vi "Ic distribution Contour_KEPCO.vi"() -> ()   [LabVIEW 2021]
uses:
  global.vi
  <vilib>/Utility/file.llb/Write Delimited Spreadsheet (DBL).vi
panel:
  in  "Field Output Channel":i32=1
  in  "NI-DAQ Device Number":i32=1
  in  "Field Read Channel":tag="Dev1/ai2"
  in  "Scale factor":dbl=34.3054
  out "Current Field mT":dbl=-2.9845698000000005
  in  "Ramp Rate V per Sec":dbl=0.001
  in  "Frequency Hz":dbl=50.0
  in  "Vmax":dbl=2.0
  out "Current Field V":dbl=-0.08700000000000002
  out "error out":errorcluster
  in  "Name":string="book14"
  in  "Contour plot folder":path=path "\\\\ad.uillinois.edu\\engr/mrl-dvh-research/Guang Yue/data/Contour plot"
  in  "End field V":dbl=-0.087 format="%#_13g"
  in  "Field step V":dbl=-0.0005 format="%#_13g"
  in  "Start field V":dbl=0.175 format="%#_13g"
  # "Set default of Ic VI before Run."
  # "Max 5mV/s"
  # "V_Field*Scale=mT"
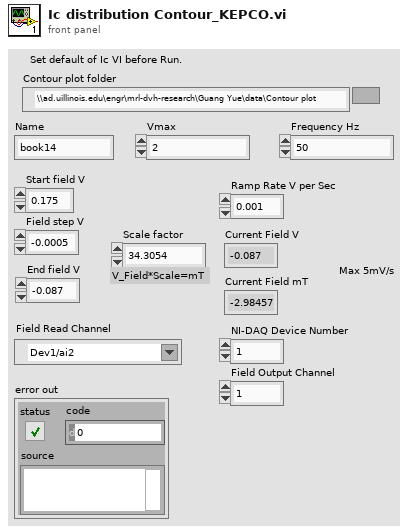
[diagram p1: front panel]
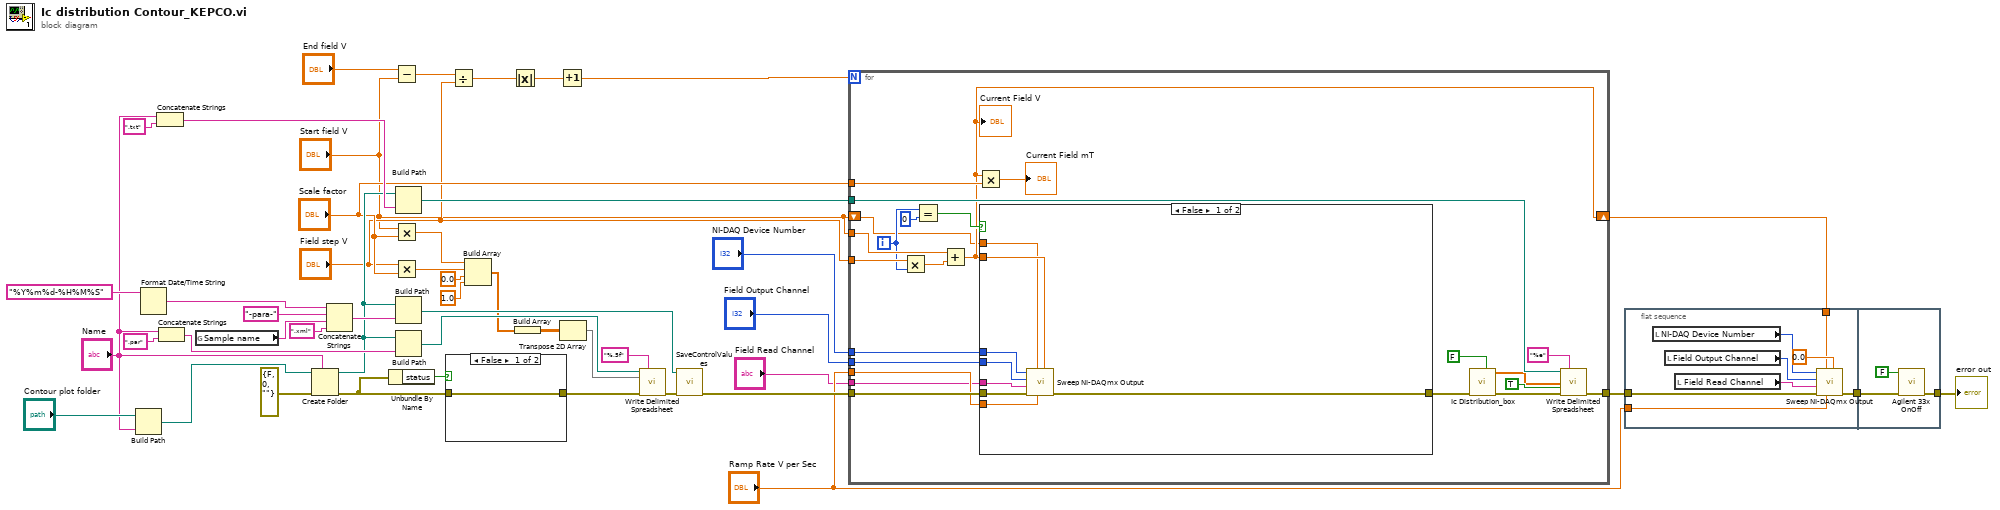
[diagram p0: block diagram]
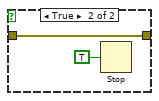
[diagram p2: hidden frame]
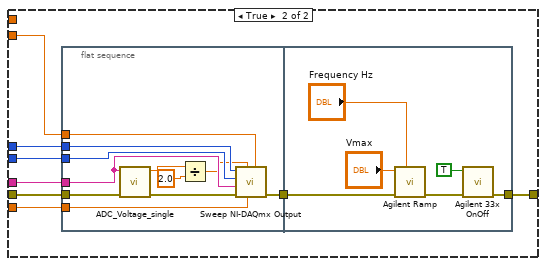
[diagram p3: hidden frame]
diagram:
  n1 = Build Path(base path="Contour plot folder", name or relative path="Name") -> (appended path=w24:path)
  n2 = Format Date/Time String(time format string (%c)="%Y%m%d-%H%M%S") -> (date/time string=w18:string)  [unwired: 2 in]
  n3 = Concatenate Strings("Name", ".txt" ("string")) -> (w28:string)
  n4 = Concatenate Strings("Name", ".par" ("string")) -> (w35:string)
  n5 = global read "global.vi" "Sample name"() -> (w17:string)
  n6 = Create Folder(prompt (Create Folder)="Name", path (use dialog)=w24, error in=errorcluster {"status"=FALSE, "code"=0, "source"=""}) -> (created path=w19:path, error out=w21:errorcluster)  [unwired: 1 out]
  n7 = Concatenate Strings(w18, "-para-" ("string"), w17, ".xml" ("string")) -> (w39:string)
  n8 = Unbundle By Name(w21) -> ("status"=w22:bool)
  n9 = Subtract(x="End field V", y="Start field V") -> (x-y=w46:dbl)
  n10 = Multiply(x="Start field V", y="Scale factor") -> (x*y=w9:dbl)
  n11 = Multiply(x="Field step V", y="Scale factor") -> (x*y=w8:dbl)
  n12 = Build Path(base path=w19, name or relative path=w28) -> (appended path=w27:path)
  n13 = Build Path(base path=w19, name or relative path=w39) -> (appended path=w37:path)
  n14 = Build Path(base path=w19, name or relative path=w35) -> (appended path=w34:path)
  n15 = case shown="False" w22 {
    tunnel: [w48 w50] -> w20
    tunnel: w21 -> [w48 w50]
    frame False {
    }
    frame True {
      n16 = Stop(stop? (T)=TRUE) -> ()
    }
  }
  n17 = Divide(x=w46, y="Field step V") -> (x/y=w45:dbl)
  n18 = Build Array(w9, w8, 0.0 ("element"), 1.0 ("element")) -> (w32:dbl[])
  n19 = Absolute Value(x=w45) -> (abs(x)=w44:dbl)
  n20 = Build Array(w32) -> (w31:dbl[][])
  n21 = Increment(x=w44) -> (x+1=w43:dbl)
  n22 = Transpose 2D Array(2D array=w31) -> (transposed array=w30:dbl[][])
  n23 = call-poly <vilib>:"Write Delimited Spreadsheet.vi"("file path (dialog if empty)"=w34, "format (%.3f)"="%.5f", "2D data"=w30, "error in (no error)"=w20) -> ("error out"=w23:errorcluster)  [unwired: 10 in, 1 out]
  n24 = call "SaveControlValues.vi"("XML File Path"=w37, "error in (no error)"=w23) -> ("error out"=w16:errorcluster)  [unwired: 8 in]
  n25 = for {
    N: w43 -> [_]
    tunnel: "Start field V" -> [w72]
    tunnel: "Field step V" -> [w71]
    tunnel: w27 -> [w66]
    tunnel: w16 -> [w64]
    tunnel: [w60] -> w15
    tunnel: "Ramp Rate V per Sec" -> [w59]
    tunnel: "Scale factor" -> [w57]
    tunnel: "Field Read Channel" -> [w56]
    tunnel: "NI-DAQ Device Number" -> [w55]
    tunnel: "Field Output Channel" -> [w54]
    shift-right: [w52] -> w1
    shift-left: "Start field V" -> [w51]
    i -> [w70]
    n26 = Multiply(x=w71, y=w70) -> (x*y=w73:dbl)
    n27 = Equal?(x=w70, y=0) -> (x = y?=w65:bool)
    n28 = Add(x=w72, y=w73) -> (x+y=w52:dbl)
    "Current Field V" <- w52
    n29 = Multiply(x=w52, y=w57) -> (x*y=→"Current Field mT":dbl)
    n30 = case shown="False" w65 {
      tunnel: w64 -> [w79 w87]
      tunnel: [w81 w86] -> w63
      tunnel: w52 -> [w80 w89]
      tunnel: w59 -> [w75 w85]
      tunnel: w56 -> [w76 w84]
      tunnel: w55 -> [w78 w83]
      tunnel: w54 -> [w77 w82]
      tunnel: w51 -> [w74 _]
      frame False {
        n31 = call "Sweep NI-DAQmx Output.vi"("Final Output Value"=w80, "Ramp Rate V/s"=w75, "Init Input Voltage"=w74, "error in"=w79, "Field Read Voltage"=w76, "Output Channel"=w77, "NI-DAQ Device Number"=w78) -> ("error out"=w81:errorcluster)  [unwired: 4 in]
      }
      frame True {
        n32 = flat-sequence {
          tunnel: w89 -> [w97]
          tunnel: [w100] -> w88
          tunnel: w87 -> [w95]
          tunnel: w85 -> [w96]
          tunnel: w84 -> [w92]
          tunnel: w83 -> [w99]
          tunnel: w82 -> [w98]
          tunnel: w88 -> [w106]
          tunnel: [w104] -> w86
          frame #0 {
            n33 = call "ADC_Voltage_single.vi"("error in"=w95, "physical channels"=w92) -> ("error out"=w94:errorcluster, "data"=w93:dbl)  [unwired: 8 in]
            n34 = Divide(x=w93, y=2.0) -> (x/y=w90:dbl)
            n35 = call "Sweep NI-DAQmx Output.vi"("Final Output Value"=w97, "Ramp Rate V/s"=w96, "Init Input Voltage"=w90, "error in"=w94, "Field Read Voltage"=w92, "Output Channel"=w98, "NI-DAQ Device Number"=w99) -> ("error out"=w100:errorcluster)  [unwired: 4 in]
          }
          frame #1 {
            n36 = call "Agilent Ramp.vi"("Frequency Hz"="Frequency Hz", "error in (no error)"=w106, "Vmax"="Vmax") -> ("error out"=w105:errorcluster)  [unwired: 8 in]
            n37 = call "Agilent 33x OnOff.vi"("error in (no error)"=w105, "Enable Output  (T: Enable)"=TRUE) -> ("error out"=w104:errorcluster)  [unwired: 9 in]
          }
        }
      }
    }
    n38 = call "Ic Distribution_box.vi"("Log Data"=FALSE, "error in no error"=w63) -> ("error out"=w61:errorcluster, "Ic array"=w62:dbl[])  [unwired: 8 in]
    n39 = call-poly <vilib>:"Write Delimited Spreadsheet.vi"("file path (dialog if empty)"=w66, "format (%.3f)"="%e", "1D data"=w62, "append to file? (new file:F)"=TRUE ("append to file? (F)"), "error in (no error)"=w61) -> ("error out"=w60:errorcluster)  [unwired: 9 in, 1 out]
  }
  n40 = flat-sequence {
    tunnel: w15 -> [w113]
    tunnel: [w114] -> w13
    tunnel: "Ramp Rate V per Sec" -> [w108]
    tunnel: w1 -> [w107]
    tunnel: [w116] -> w14
    tunnel: w13 -> [w117]
    frame #0 {
      n41 = local read "NI-DAQ Device Number"() -> (w112:i32)
      n42 = local read "Field Output Channel"() -> (w111:i32)
      n43 = local read "Field Read Channel"() -> (w110:tag)
      n44 = call "Sweep NI-DAQmx Output.vi"("Final Output Value"=0.0, "Ramp Rate V/s"=w108, "Init Input Voltage"=w107, "error in"=w113, "Field Read Voltage"=w110, "Output Channel"=w111, "NI-DAQ Device Number"=w112) -> ("error out"=w114:errorcluster)  [unwired: 4 in]
    }
    frame #1 {
      n45 = call "Agilent 33x OnOff.vi"("error in (no error)"=w117, "Enable Output  (T: Enable)"=FALSE) -> ("error out"=w116:errorcluster)  [unwired: 9 in]
    }
  }
  "error out" <- w14
